vi "CalcSummaryUncertainties.vi"(8 "error in (no error)":errorcluster, 10 "Limits":dbl[][][](array[numeric]), 11 "Uncertainties":dbl[][][](array[numeric]) format="%.6f") -> (0 "error out":errorcluster, 3 "PFI":string[][][](array[string]))   [LabVIEW 2014]
uses:
  typedef/PMUConfig.ctl
panel:
  in  "Tab Control":enum32{"Uncertainties", "Limits", "PFI"}(tab)
  # "V+ TVE"
  # "I+ TVE"
  # "VA TVE"
  # "VB TVE"
  # "VC TVE"
  # "IA TVE"
  # "IB TVE"
  # "IC TVE"
  # "Freq Hz"
  # "ROCOF HZ/s"
  # "FreqRng"
  # "MagRng"
  # "Harmonics"
  # "Out-of-Band"
  # "Amplitude Mod"
  # "Phase Mod"
  # "FreqRamp +"
  # "FreqRamp -"
  # "VA TVE"
  # "VB TVE"
  # "VC TVE"
  # "V+ TVE"
  # "IA TVE"
  # "IB TVE"
  # "IC TVE"
  # "I+ TVE"
  # "FE"
  # "RFE"
  # "FreqRng"
  # "MagRng"
  # "Harm"
  # "OOB"
  # "Phase Mod"
  # "Ampl Mod"
  # "Freq Ramp +"
  # "Freq Ramp -"
  # "FreqRng"
  # "MagRng"
  # "Harm"
  # "OOB"
  # "Phase Mod"
  # "Ampl Mod"
  # "Freq Ramp +"
  # "Freq Ramp -"
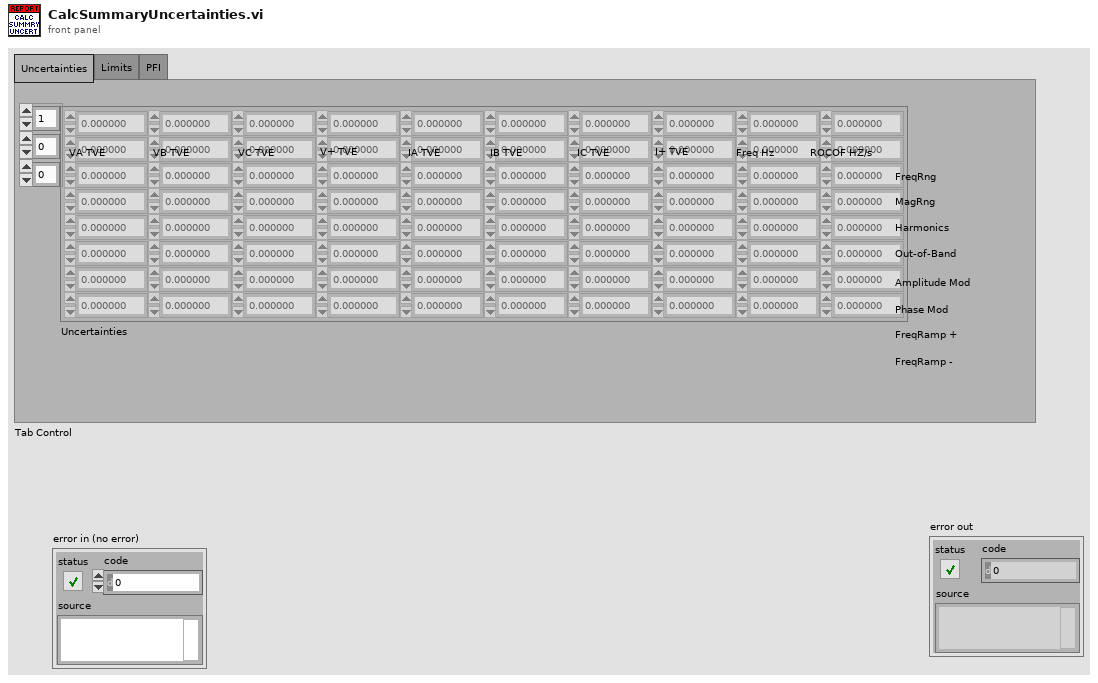
[diagram p1: front panel]
types:
  T1 = typedef "PMUConfig.ctl" = cluster{"Class":string, "Fs":dbl, "F0":dbl}
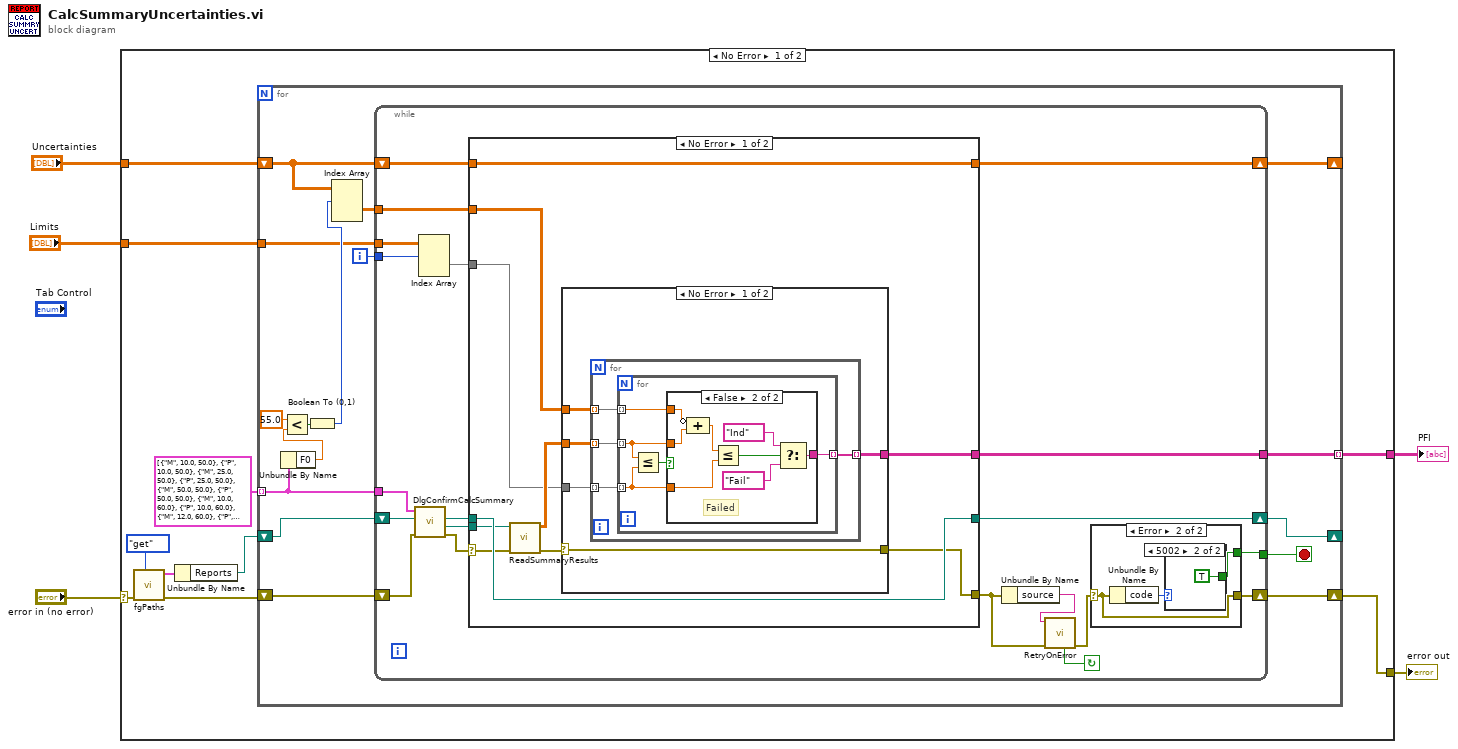
[diagram p0: block diagram]
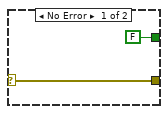
[diagram p2: hidden frame]
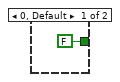
[diagram p3: hidden frame]
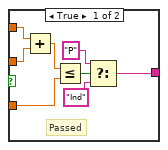
[diagram p4: hidden frame]
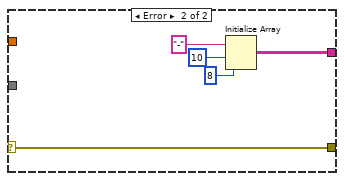
[diagram p5: hidden frame]
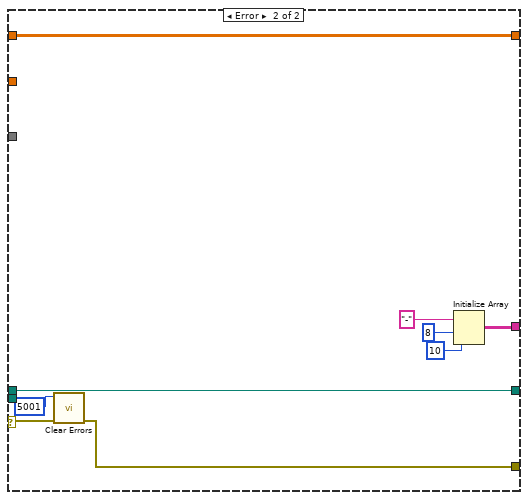
[diagram p6: hidden frame]
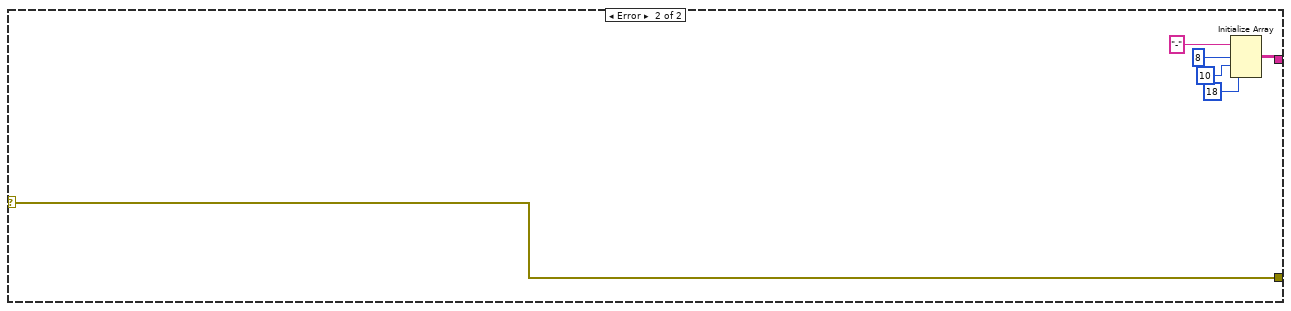
[diagram p7: hidden frame]
diagram:
  n1 = case shown="No Error" "error in (no error)" {
    selector: "error in (no error)" -> [w9 w118]
    tunnel: [w14 w118] -> w4
    tunnel: "Uncertainties" -> [w12 _]
    tunnel: [w13 w114] -> w2
    tunnel: "Limits" -> [w11 _]
    frame No Error {
      n2 = call "fgPaths.vi"("cmd"=enum16{"init", "set", "get"}."get", "error in (no error)"=w9) -> ("error out"=w8:errorcluster, "clPaths"=w10:cluster{"Templates":path, "Reports":path})  [unwired: 8 in]
      n3 = Unbundle By Name(w10) -> ("Reports"=w7:path)
      n4 = for {
        tunnel: T1[] [{"Class"="M", "Fs"=10.0, "F0"=50.0}, {"Class"="P", "Fs"=10.0, "F0"=50.0}, {"Class"="M", "Fs"=25.0, "F0"=50.0}, {"Class"="P", "Fs"=25.0, "F0"=50.0}, {"Class"="M", "Fs"=50.0, "F0"=50.0}, {"Class"="P", "Fs"=50.0, "F0"=50.0}, {"Class"="M", "Fs"=10.0, "F0"=60.0}, {"Class"="P", "Fs"=10.0, "F0"=60.0}, {"Class"="M", "Fs"=12.0, "F0"=60.0}, {"Class"="P", "Fs"=12.0, "F0"=60.0}, {"Class"="M", "Fs"=15.0, "F0"=60.0}, {"Class"="P", "Fs"=15.0, "F0"=60.0}, {"Class"="M", "Fs"=20.0, "F0"=60.0}, {"Class"="P", "Fs"=20.0, "F0"=60.0}, {"Class"="M", "Fs"=30.0, "F0"=60.0}, {"Class"="P", "Fs"=30.0, "F0"=60.0}, {"Class"="M", "Fs"=60.0, "F0"=60.0}, {"Class"="P", "Fs"=60.0, "F0"=60.0}] -> [w23] mode=indexing
        shift-right: [w28] -> w14
        shift-left: w8 -> [w30]
        shift-right: [w27] -> _
        shift-left: w12 -> [w24]
        shift-right: [w26] -> _
        shift-left: w7 -> [w31]
        tunnel: [w25] -> w13 mode=indexing
        tunnel: w11 -> [w17]
        i -> [w16]
        stop <- w29 stop-if-true
        n5 = Unbundle By Name(w23) -> ("F0"=w22:dbl)
        n6 = Less?(x=55.0, y=w22) -> (x < y?=w20:bool)
        n7 = Boolean To (0,1)(Boolean=w20) -> (0, 1=w19:i16)
        n8 = Index Array(array=w24, index (dim 0)=w19) -> (element=w18:dbl[][])  [unwired: 2 in]
        n9 = while {
          tunnel: w23 -> [w51]
          tunnel: [w37] -> w29
          shift-right: [w43] -> w26
          shift-left: w31 -> [w50]
          shift-right: [w38] -> w28
          shift-left: w30 -> [w49]
          shift-right: [w46] -> w27
          shift-left: w24 -> [w47]
          tunnel: [w36] -> w25
          tunnel: w18 -> [w35]
          tunnel: w17 -> [w34]
          tunnel: w16 -> [w32]
          stop <- w42 continue-if-true
          n10 = call "DlgConfirmCalcSummary.vi"("error in (no error)"=w49, "Path"=w50, "PMUConfig"=w51) -> ("error out"=w48:errorcluster, "Summary Data Excel File"=w45:path, "Path"=w44:path)  [unwired: 5 in, 1 out]
          n11 = Index Array(array=w34, index (dim 0)=w32) -> (element=w33:dbl[][])  [unwired: 2 in]
          n12 = case shown="No Error" w48 {
            selector: w48 -> [w67 w112]
            tunnel: [w65 w111] -> w41
            tunnel: w47 -> [w61 w109]
            tunnel: [w61 w109] -> w46
            tunnel: w45 -> [w66 _]
            tunnel: w44 -> [w68 w108]
            tunnel: [w68 w108] -> w43
            tunnel: [w63 w104] -> w36
            tunnel: w35 -> [w62 _]
            tunnel: w33 -> [w60 _]
            frame No Error {
              n13 = call "ReadSummaryResults.vi"("error in (no error)"=w67, "Path"=w66) -> ("error out"=w59:errorcluster, "Results"=w64:dbl[][])  [unwired: 8 in]
              n14 = case shown="No Error" w59 {
                selector: w59 -> [w73 w103]
                tunnel: [w73 w103] -> w65
                tunnel: w60 -> [w70 _]
                tunnel: w62 -> [w71 _]
                tunnel: w64 -> [w72 _]
                tunnel: [w69 w99] -> w63
                frame No Error {
                  n15 = for {
                    tunnel: w72 -> [w76] mode=indexing
                    tunnel: w71 -> [w75] mode=indexing
                    tunnel: w70 -> [w77] mode=indexing
                    tunnel: [w74] -> w69 mode=indexing
                    n16 = for {
                      tunnel: w77 -> [w80] mode=indexing
                      tunnel: w76 -> [w79] mode=indexing
                      tunnel: w75 -> [w81] mode=indexing
                      tunnel: [w78] -> w74 mode=indexing
                      n17 = Less Or Equal?(x=w79, y=w80) -> (x <= y?=w82:bool)
                      n18 = case shown="False" w82 {
                        tunnel: w81 -> [w90 w98]
                        tunnel: w80 -> [w87 w95]
                        tunnel: w79 -> [w89 w97]
                        tunnel: [w83 w91] -> w78
                        frame True {
                          # "Passed"
                          n19 = Add(x=w90, y=w89) -> (x+y=w88:dbl)
                          n20 = Less Or Equal?(x=w88, y=w87) -> (x <= y?=w86:bool)
                          n21 = Select(t="P", s=w86, f="Ind") -> (s? t:f=w83:string)
                        }
                        frame False {
                          # "Failed"
                          n22 = Compound Arithmetic op=ADD(invert w98, w97) -> (w96:dbl)
                          n23 = Less Or Equal?(x=w96, y=w95) -> (x <= y?=w94:bool)
                          n24 = Select(t="Ind", s=w94, f="Fail") -> (s? t:f=w91:string)
                        }
                      }
                    }
                  }
                }
                frame Error {
                  n25 = Initialize Array("-", 10 ("dimension size"), 8 ("dimension size")) -> (w99:string[][])
                }
              }
            }
            frame Error {
              n26 = call <vilib>:"Clear Errors.vi"("error in (no error)"=w112, "specific error code to clear (0: all)"=5001) -> ("error out"=w111:errorcluster)  [unwired: 4 in, 1 out]
              n27 = Initialize Array("-", 8 ("dimension size"), 10 ("dimension size")) -> (w104:string[][])
            }
          }
          n28 = Unbundle By Name(w41) -> ("source"=w40:string)
          n29 = call "RetryOnError.vi"("error in (no error)"=w41, "Error Msg"=w40) -> ("error out"=w39:errorcluster, "Retry"=w42:bool)  [unwired: 8 in]
          n30 = case shown="Error" w39 {
            selector: w39 -> [w53 w54]
            tunnel: [w53 w54] -> w38
            tunnel: [FALSE w55] -> w37
            frame No Error {
            }
            frame Error {
              n31 = Unbundle By Name(w54) -> ("code"=w56:i32)
              n32 = case shown="5002" w56 {
                tunnel: [FALSE TRUE] -> w55
                frame 0, Default {
                }
                frame 5002 {
                }
              }
            }
          }
        }
      }
    }
    frame Error {
      n33 = Initialize Array("-", 8 ("dimension size"), 10 ("dimension size"), 18 ("dimension size")) -> (w114:string[][][])
    }
  }
  "error out" <- w4
  "PFI" <- w2
